vi "ReadNet_Torch.vi"(8 "error in":errorcluster, 9 "evaluate":bool=TRUE, 10 "isBinary":bool=TRUE, 11 "ModelPath":path) -> (0 "error out":errorcluster, 3 "NET":refnum<class "NET.lvclass">)   [LabVIEW 2020, in "OpenLvVision_OpenCv.lvlib"]
doc: "Reads a network model stored in Torch7 framework's format."
uses:
  OpenLvVision_OpenCv.lvlib
  NET/NET.lvclass
  _LvHelpers/EdvrObject/TypeDef/Edvr.ctl
  _LvHelpers/EdvrObject/EdvrObject.lvclass
  Dlls/OlvOpenCvWrapper.dll
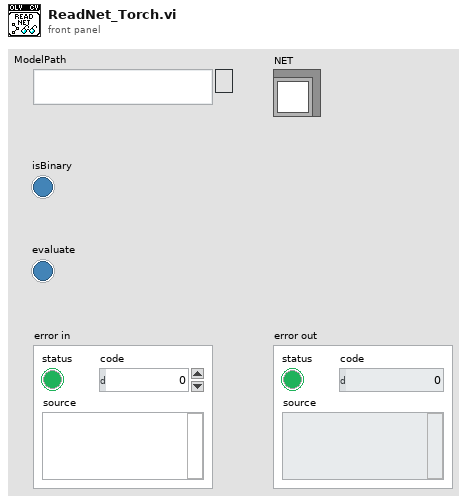
[diagram p1: front panel]
types:
  T1 = typedef "OpenLvVision_OpenCv.lvlib/EdvrObject.lvclass/Edvr.ctl" = refnum<data-value>
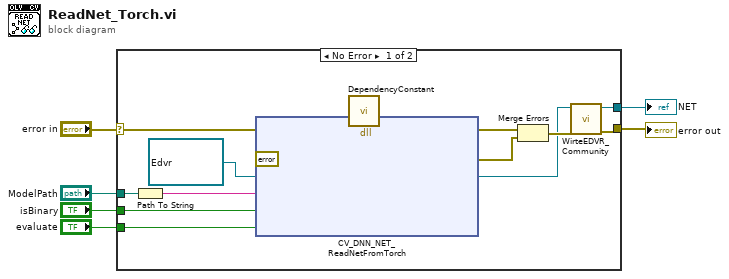
[diagram p0: block diagram]
diagram:
  n1 = case shown="No Error" "error in" {
    selector: "error in" -> [w16 w20]
    tunnel: [w14 w20] -> w5
    tunnel: [w12 _] -> w4
    tunnel: "ModelPath" -> [w11 _]
    tunnel: "isBinary" -> [w8 _]
    tunnel: "evaluate" -> [w7 _]
    frame No Error {
      n2 = Path To String(path=w11) -> (string=w10:string)
      n3 = dll-call lib="C:/Users/lukas/Downloads/OpenLvVision_OpenCv/SourceCode/LabView/OpenLvVision_OpenCv/Dlls/OlvOpenCvWrapper.dll" fn="CV_DNN_NET_ReadNetFromTorch"(error in=w16, "Error"=errorcluster {"status"=FALSE, "code"=0, "source"=""} ("error out"), "edvrRef"=T1 refnum ("Edvr"), "modelPath"=w10, "isBinary"=w8, "evaluate"=w7) -> (error out=w19:errorcluster, "Error"=w18:errorcluster, "edvrRef"=w13:T1)  [unwired: 6 in, 1 out]
      n4 = call "DependencyConstant.vi"() -> ()  [unwired: 12 in]
      n5 = Merge Errors(w19, w18) -> (w15:errorcluster)
      n6 = call "WirteEDVR_Community.vi"("error in"=w15, "Edvr"=w13) -> ("error out"=w14:errorcluster, "NET"=w12:refnum<class "NET.lvclass">)  [unwired: 8 in]
    }
    frame Error {
    }
  }
  "NET" <- w4
  "error out" <- w5
